vi "basement tank 1.vi"() -> ()   [LabVIEW 2019]
uses:
  <vilib>/NI/Current Value Table/Type Defs/Single Tag.ctl
  <vilib>/NI/Current Value Table/Type Defs/Data Types.ctl
  <vilib>/Utility/miscctls.llb/LVPointTypeDef.ctl
  <vilib>/NI/STM/TCP/Read Meta Data (TCP Ref).vi
  <vilib>/NI/STM/TCP/Get Connection Reference (TCP).vi
  <vilib>/NI/AMC/Read Termination Message.vi
  <vilib>/NI/AMC/Create Single Message.vi
  <vilib>/NI/AMC/Update Message Routing Info.vi
  <vilib>/NI/STM/TCP/Read Meta Data (TCP Clst).vi
  <vilib>/NI/AMC/Globals.vi
  <vilib>/NI/STM/TCP/Write Message (TCP).vi
  <vilib>/NI/AMC/Send Message.vi
  <vilib>/NI/AMC/AMC.lvlib
  <vilib>/NI/STM/NI STM.lvlib
  <vilib>/NI/Current Value Table/Current Value Table.lvlib
panel:
  in  "Auto Level Main Tank":dbl(knob)=250.0 min=250.0 max=950.0 step=1.0 scale=200.0..1000.0 scale format="%#.3g"
  in  "Enable DI Auto Top-up":bool
  in  "Sulfuric Proc 1":dbl=2.0 caption="ml Acid Proc 1" min=0.0 max=5000.0 step=1.0
  in  "Trig Sulfuric Proc1":bool caption="Trigger Dose"
  out "Flow":bool
  in  "LEV Proc 1":dbl=2.0 caption="ml Lev Proc 1" min=0.0 max=1000.0 step=1.0
  in  "Trig Level Proc1":bool caption="Trigger Dose"
  in  "UCON Proc 1":dbl=2.0 caption="ml UCON Proc 1" min=0.0 max=1000.0 step=1.0
  in  "Trig UCON Proc 1":bool caption="Trigger Dose"
  in  "SPS Proc 1":dbl=2.0 caption="ml SPS Proc 1" min=0.0 max=1000.0 step=1.0
  in  "Trig SPS Proc 1":bool caption="Trigger Dose"
  in  "BasT1_Level Last Hr":bool
  in  "BasT1_Flow Last Hr":bool
  in  "Specific Gravity":dbl(knob)=1.0 min=1.0 max=1.25 step=0.0025 scale=1.0..1.25
  in  "CuOAddAmount":dbl caption="CuO grams to add" min=-1000.0 max=1000.0 step=1.0
  out "Grams CuO to Add":dbl format="%.1f"
  in  "Dose Extra Oxide":bool
  out "BTnk1 SG":dbl format="%.3f"
  in  "FlowInd OxSys":dbl(slide) scale=0.0..15.0
  out "Chilled Injection":u8(slide) scale=0.0..100.0
  out "Tempered Injection":u8(slide) scale=0.0..100.0
  in  "BasT1_P Last Hr":bool
  in  "BasT1_T Last Hr":bool
  out "Boiler Water Facilities Valve":dbl(slide) scale=0.0..100.0
  out "Tempered Water Facilities Valve":dbl(slide) scale=0.0..100.0
  out "Chilled Water Facilities Valve":dbl(slide) scale=0.0..100.0
  out "Boiler Water Out":dbl(knob) scale=10.0..110.0
  out "Boiler Water In":dbl(knob) scale=10.0..110.0
  out "Tempered Water Out":dbl(knob) scale=10.0..35.0
  out "Tempered Water In":dbl(knob) scale=10.0..35.0
  out "Chilled Water Out":dbl(knob) scale=0.0..25.0
  out "Chilled Water In":dbl(knob) scale=0.0..25.0
  out "E Stop":bool
  out "OxideToFilter":bool
  out "Oxide Pump":bool
  out "Boolean 4":bool
  out "OxideDose Indicate":bool
  out "To Plating Process 1 & 2":bool
  out "ThreewayLowerElbow":bool
  in  "Tab Control":enum32{"Main Pump", "Lift Pump"}(tab)
  out "Amps":dbl format="%#.2g"
  out "Volts":dbl format="%#.1f"
  out "VFD T":dbl format="%#.2g"
  out "RPM":dbl format="%#.2f"
  out "Fault Code":dbl format="%#.2g"
  out "Freq":dbl format="%#.2g"
  out "PipeToTank":bool
  out "Tnk1Tee 2":bool
  out "Boolean 6":bool
  out "Circulator":bool
  out "Run Enabled?":bool
  out "Supply Pressure (kPa)":dbl(knob) scale=0.0..250.0
  out "Supply Temperature":dbl(slide) scale=0.0..100.0
  in  "Draining System to Tree":bool
  in  "Liters DI to Add":dbl(knob) min=0.0 max=500.0 step=1.0 scale=0.0..500.0
  in  "Add DI Water":bool
  out "PipeToPump 2":bool
  out "Total Added":dbl format="%.2g"
  out "DI Flow (L/min)":dbl(knob) scale=0.0..100.0
  out "Total Flow (when operated with plating tanks)":dbl(knob) scale=0.0..150.0
  in  "Flow to Reactor (L/min)":dbl(knob)=5.0 min=5.0 max=20.0 step=0.1 scale=5.0..12.0 scale format="%#.1g"
  in  "Enable Oxide Reactor":bool
  in  "Enable T-Control":bool
  in  "Temperature Setpoint":dbl(knob) step=0.1 scale=12.0..30.0 scale format="%#.1g"
  in  "Supply Pressure (kPa)":dbl(knob)=50.0 min=50.0 max=200.0 step=5.0 scale=50.0..200.0
  out "HeatExchanger":bool
  out "PipeToPump":bool
  out "Tnk1Tee":bool
  in  "Enable Main Pump":bool
  out "Main Pump":bool
  out "Tank":dbl(slide) scale=0.0..1000.0
  in  "Machine":bool
  in  "Basement 4":bool
  in  "Dryer":bool
  in  "Rinse 4":bool
  in  "Rinse 3":bool
  in  "Rinse 2":bool
  in  "Basement 3":bool
  in  "Basement 2":bool
  in  "Basement 1":bool
  in  "Plater 6":bool
  in  "Plater 5":bool
  in  "Plater 4":bool
  in  "Plater 3":bool
  in  "Plater 2":bool
  in  "Plater 1":bool
  in  "Predip":bool
  in  "Rinse 1":bool
  in  "Cleaner":bool
  in  "Etch":bool
  out "status":string
  # "Module Selection"
  # "@"
  # "SG"
  # "Dosing"
  # "SPS"
  # "UCON"
  # "Leveler"
  # "Sulfuric Acid"
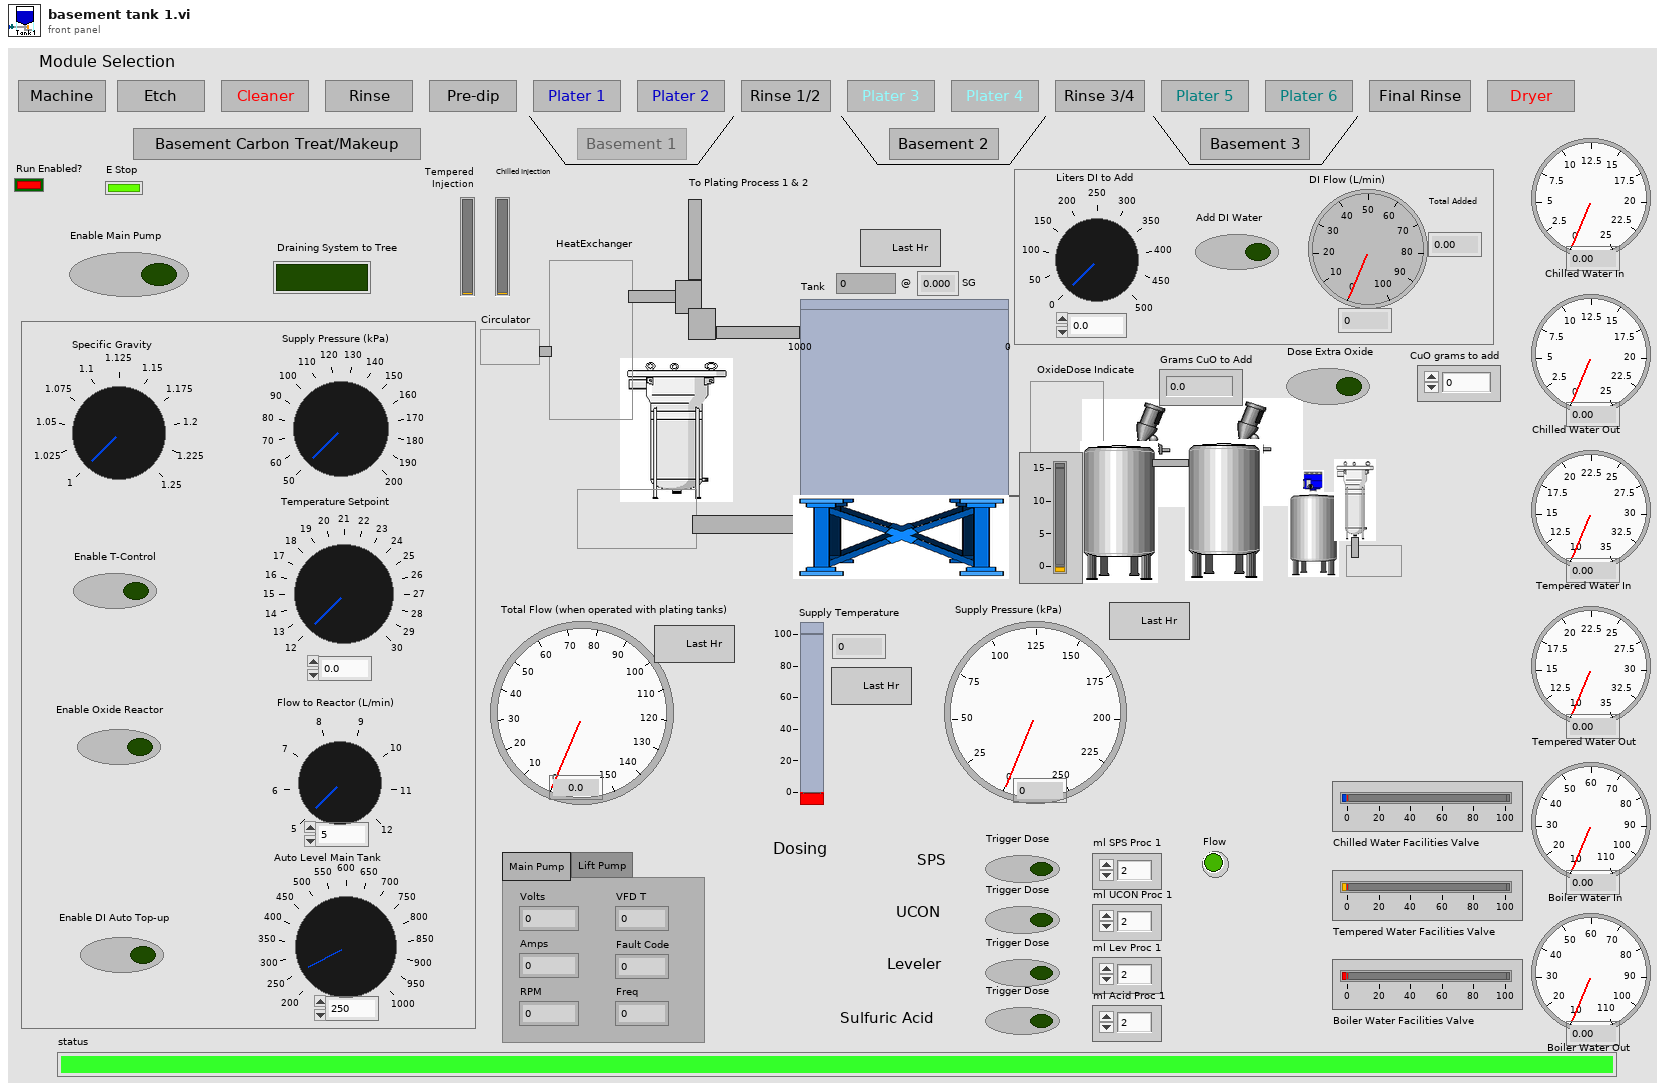
[diagram p1: front panel]
types:
  T1 = typedef "Current Value Table.lvlib/Single Tag.ctl" = cluster{"Data Type":T2, "Name":string, "Value":string, "Description":string}
  T2 = typedef "Current Value Table.lvlib/Data Types.ctl" = enum16{"Double", "Single", "I64", "I32", "I16", "I8", "U64", "U32", "U16", "U8", "String", "Boolean", "Array of U8", "Array of U16", "Array of U32", "Array of U64", "Array of I64", "Array of I32", "Array of I16", "Array of I8", "Array of Double", "Array of Single", "Array of Boolean", "Array of String"}
  T3 = typedef "NI STM.lvlib/TCP Connection Info.ctl" = cluster{"connection ID":refnum<k5>, "meta data":T4[]}
  T4 = typedef "NI STM.lvlib/MetaDataElement.ctl" = string
  T5 = typedef "AMC.lvlib/Message Queue.ctl" = refnum<queue>
  T6 = cluster{"Shift":bool, "Ctrl":bool, "Alt":bool, "Cmd":bool, "Opt":bool}
  T7 = enum8{"Enabled", "Disabled", "Disabled and Grayed Out"}
  T8 = typedef "LVPointTypeDef.ctl" = cluster{"Horizontal":i16, "Vertical":i16}
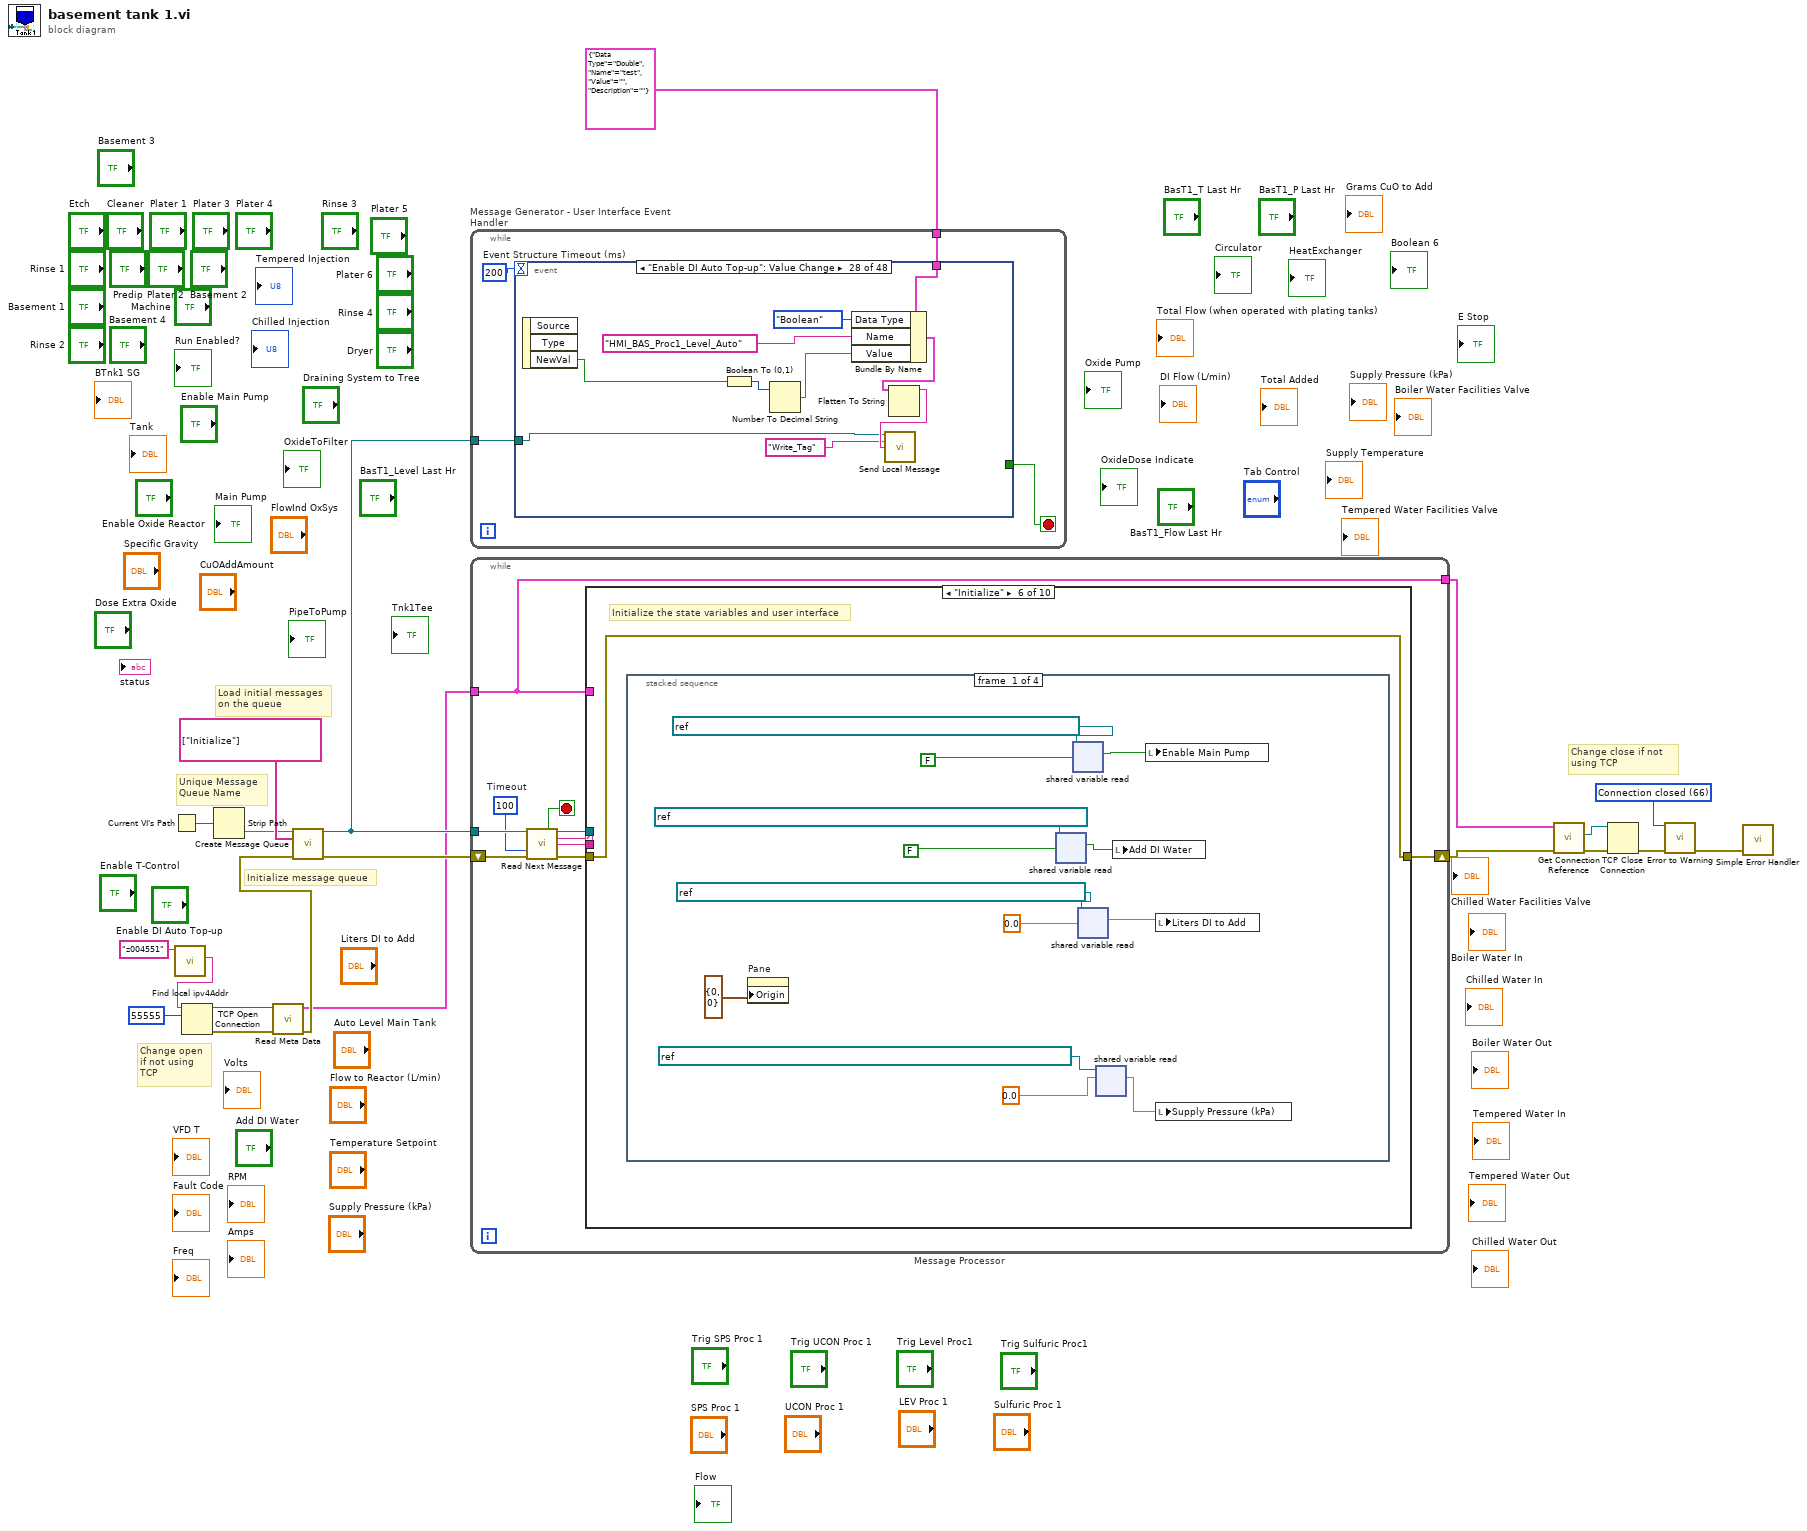
[diagram p0: block diagram]
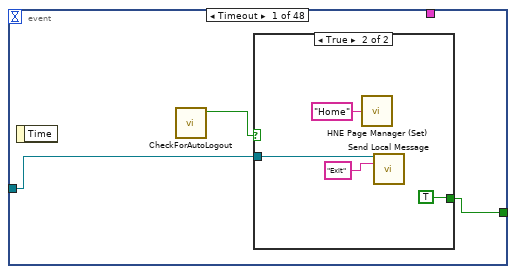
[diagram p2: hidden frame]
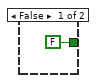
[diagram p3: hidden frame]
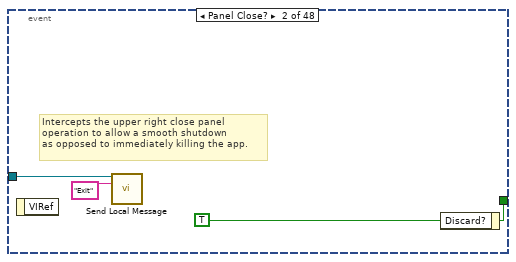
[diagram p4: hidden frame]
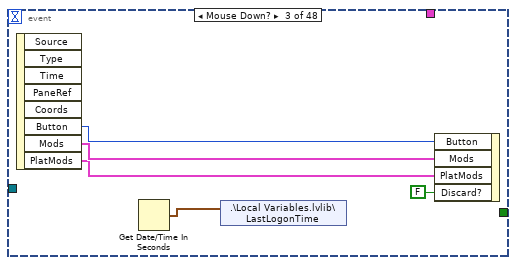
[diagram p5: hidden frame]
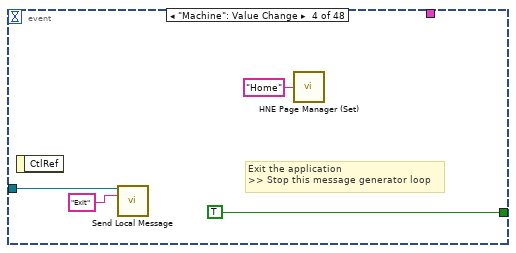
[diagram p6: hidden frame]
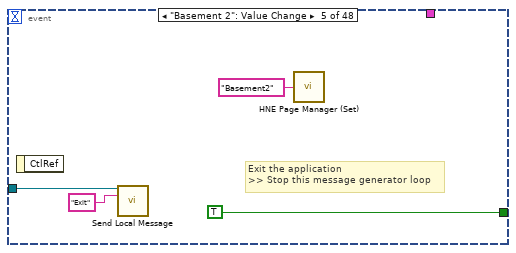
[diagram p7: hidden frame]
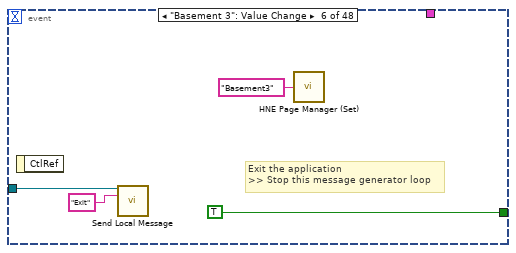
[diagram p8: hidden frame]
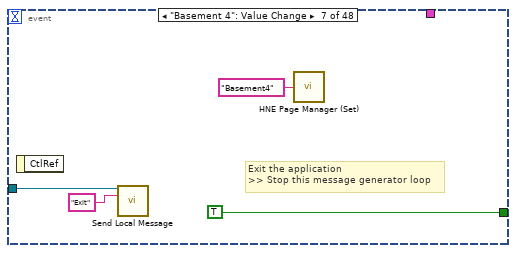
[diagram p9: hidden frame]
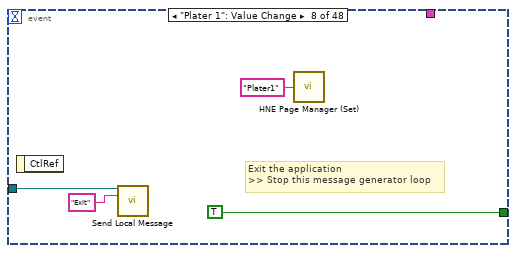
[diagram p10: hidden frame]
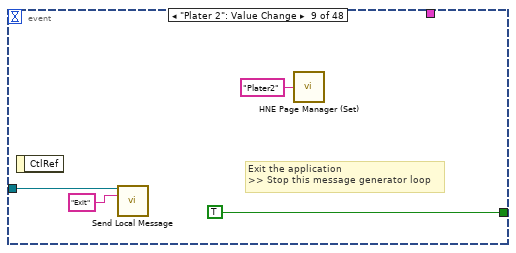
[diagram p11: hidden frame]
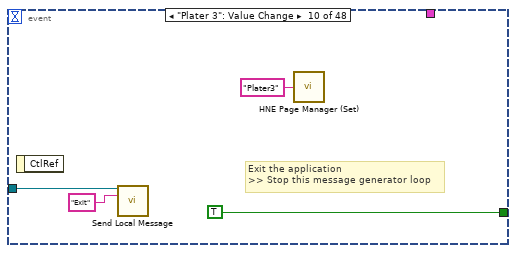
[diagram p12: hidden frame]
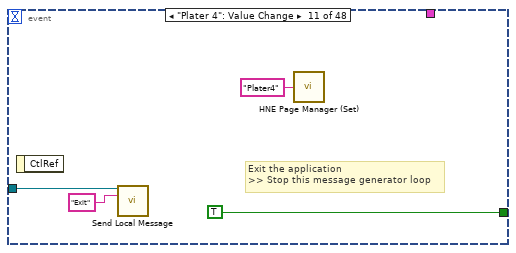
[diagram p13: hidden frame]
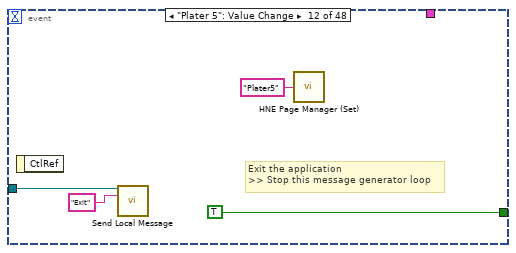
[diagram p14: hidden frame]
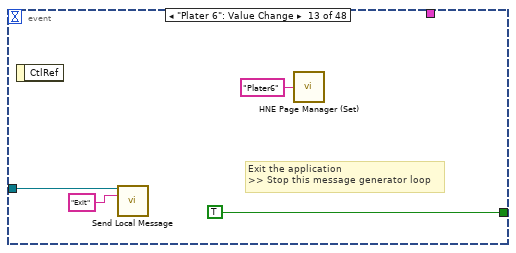
[diagram p15: hidden frame]
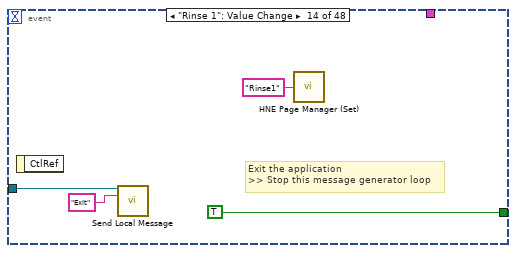
[diagram p16: hidden frame]
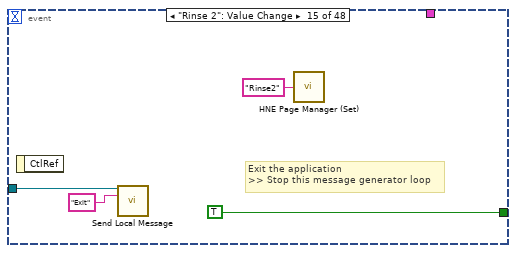
[diagram p17: hidden frame]
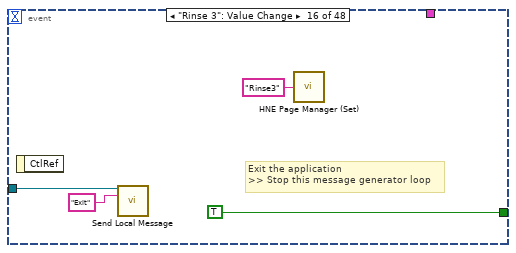
[diagram p18: hidden frame]
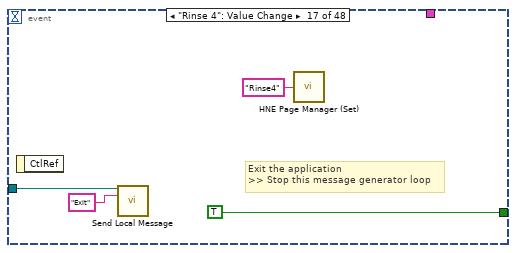
[diagram p19: hidden frame]
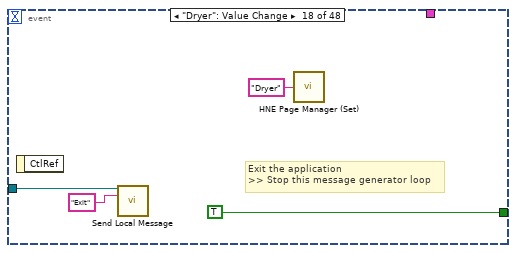
[diagram p20: hidden frame]
diagram:
  w9 = 66 items=["No Error", "Argument Error", "Memory Full", "Out of Zone", "End of File", "File Already Open", "Generic File IO Error", "File Not Found", "File Permission Error", "Disk Full", "Duplicate Path", "Too Many Files Open", "Not Enabled", "Resource File Not Found", "Cannot Add Resource", "Resource Not Found", "Image Not Found", "Image Memory Error", "Pen Does Not Exist", "Config Bad Type", "Config Token Not Found", "Config Parse Error", "Config Memory Error", "Bad External Code Format", "Bad External Code Offset", "External Code Not Present", "Null Window", "Destroy Window Mixup", "Null Menu", "Print Aborted", "Bad Print Record", "Print Driver Error", "Windows Error During Print", "Memory Error During Print", "Print Dialog Error", "Generic Print Error", "Invalid Device Refnum", "Device Not Found", "Device Parameter Error", "Device Unit Error", "Can't Open Device", "Device Call Aborted", "Generic Error", "Cancelled By User", "Object ID Too Low", "Object ID Too High", "Object Not In Heap", "Unknown Heap", "Bad DefProc ID", "DefProc Not In Table", "Message Out Of Range", "Null Method", "Unknown Message", "Manager Call Not Supported", "Bad address", "Connection In progress", "Connection timed out", "Connection is already in progress", "Network attribute not supported", "Network error", "Address in use", "System out of memory", "Connection aborted", "Connection refused", "Connection is not connected", "Connection is already connected", "Connection closed", "Initialize error (interapplication manager)", "Bad occurrence", "Wait on unbound occurrence handler", "Occurrence queue overflow", "Bad path", "Semaphore not signaled", "Unrecognized type (interapplication manager)"] ("1st Error to Convert")
  # "Change close if not using TCP"
  # "Change open if not using TCP"
  # "Initialize message queue"
  # "Unique Message\nQueue Name"
  # "Load initial messages\non the queue"
  n1 = Current VI's Path() -> (path=w16:path)
  n2 = call "Find local ipv4Addr.vi"("MachineToFind"="z004551" ("Target IP Address")) -> ("name"=w1:string)  [unwired: 9 in, 1 out]
  n3 = TCP Open Connection(address=w1, remote port or service name=u16 55555 ("remote port")) -> (connection ID=w14:refnum<k5>, error out=w13:errorcluster)  [unwired: 1 in, 2 out]
  n4 = Strip Path(path=w16) -> (name=w19:string)  [unwired: 1 out]
  n5 = call-poly <vilib>:"Read Meta Data.vi"("error in"=w13, "connection ID"=w14) -> ("error out"=w12:errorcluster, "connection info out"=w11:T3)  [unwired: 7 in, 1 out]
  n6 = call <vilib>:"Create Message Queue.vi"("message queue name"=w19, "initial message names"=string[] ["Initialize"], "error in"=w12) -> ("message queue out"=w18:T5, "error out"=w17:errorcluster)  [unwired: 11 in]
  n7 = while "Message Generator - User Interface Event Handler" {
    tunnel: w18 -> [w22]
    tunnel: T1 {"Data Type"=enum."Double", "Name"="test", "Value"="", "Description"=""} ("Tag") -> [w21]
    stop <- w23 stop-if-true
    w24 = 200  # Event Structure Timeout (ms)
    n8 = event shown="[27] \"Enable DI Auto Top-up\": Value Change" {
      selector: _ -> [_ _ _ _ _ _ _ _ _ _ _ _ _ _ _ _ _ _ _ _ _ _ _ _ _ _ _ _ _ _ _ _ _ _ _ _ _ _ _ _ _ _ _ _ _ _ _ _]
      dyn-events: _ -> [_ _ _ _ _ _ _ _ _ _ _ _ _ _ _ _ _ _ _ _ _ _ _ _ _ _ _ _ _ _ _ _ _ _ _ _ _ _ _ _ _ _ _ _ _ _ _ _]
      timeout: w24 -> [_ _ _ _ _ _ _ _ _ _ _ _ _ _ _ _ _ _ _ _ _ _ _ _ _ _ _ _ _ _ _ _ _ _ _ _ _ _ _ _ _ _ _ _ _ _ _ _]
      tunnel: [w25 w35 _ TRUE ("Discard?") TRUE ("Discard?") TRUE ("Discard?") TRUE ("Discard?") TRUE ("Discard?") TRUE ("Discard?") TRUE ("Discard?") TRUE ("Discard?") TRUE ("Discard?") TRUE ("Discard?") TRUE ("Discard?") TRUE ("Discard?") TRUE ("Discard?") TRUE ("Discard?") TRUE ("Discard?") TRUE ("Discard?") TRUE ("Discard?") TRUE ("Discard?") _ _ _ _ _ _ _ _ _ _ _ _ _ _ _ _ _ _ _ _ _ _ _ _ _ _ _] -> w23
      tunnel: w22 -> [w26 w33 _ w42 w46 w50 w54 w58 w62 w66 w70 w74 w78 w82 w86 w90 w94 w98 w102 w106 w110 w113 w115 w125 w135 w145 w155 w165 w175 w185 w195 w205 w215 w225 w234 w243 w252 w261 w270 w279 w288 w297 w306 w315 w324 w329 w334 w339]
      tunnel: w21 -> [_ _ _ _ _ _ _ _ _ _ _ _ _ _ _ _ _ _ _ _ _ _ w116 w126 w136 w146 w156 w166 w176 w186 w196 w206 w216 w228 w237 w246 w255 w264 w273 w282 w291 w300 w309 w318 _ _ _ _]
      event Timeout {
        n9 = event-data() -> ()  [unwired: 2 out]
        n10 = call "CheckForAutoLogout.vi"() -> ("Boolean"=w27:bool)  [unwired: 11 in]
        n11 = case shown="True" w27 {
          tunnel: [FALSE ("Discard?") TRUE ("Discard?")] -> w25
          tunnel: w26 -> [_ w29]
          frame False {
          }
          frame True {
            n12 = call <userlib>:"HNE Page Manager (Set).vi"("Next Page"="Home") -> ()  [unwired: 4 in, 1 out]
            n13 = call <vilib>:"Send Local Message.vi"("message queue in"=w29, "message name"="Exit") -> ()  [unwired: 11 in, 3 out]
          }
        }
      }
      event Panel Close? {
        w35 = TRUE ("Discard?")
        # "Intercepts the upper right close panel\noperation to allow a smooth shutdown\nas opposed to immediately killing the app."
        n14 = event-data() -> ()  [unwired: 2 out]
        n15 = call <vilib>:"Send Local Message.vi"("message queue in"=w33, "message name"="Exit") -> ()  [unwired: 11 in, 3 out]
        n16 = event-data("Discard?"=w35) -> ()  [unwired: 1 in, 1 out]
      }
      event Mouse Down? {
        n17 = event-data() -> ("Button"=w40:u16, "Mods"=w39:cluster{"Double Click":bool, "Menu Key":bool}, "PlatMods"=w38:T6)  [unwired: 6 out]
        n18 = Get Date/Time In Seconds() -> (seconds since 1Jan1904=w36:timestamp)
        n19 = shared-variable ".\\Local Variables.lvlib\\LastLogonTime"(w36) -> ()  [unwired: 1 in, 1 out]
        n20 = event-data("Button"=w40, "Mods"=w39, "PlatMods"=w38, "Discard?"=FALSE) -> ()  [unwired: 1 in, 1 out]
      }
      event "Machine": Value Change {
        # "Exit the application\n>> Stop this message generator loop"
        n21 = event-data() -> ()  [unwired: 2 out]
        n22 = call <vilib>:"Send Local Message.vi"("message queue in"=w42, "message name"="Exit") -> ()  [unwired: 11 in, 3 out]
        n23 = call <userlib>:"HNE Page Manager (Set).vi"("Next Page"="Home") -> ()  [unwired: 4 in, 1 out]
      }
      event "Basement 2": Value Change {
        # "Exit the application\n>> Stop this message generator loop"
        n24 = event-data() -> ()  [unwired: 2 out]
        n25 = call <vilib>:"Send Local Message.vi"("message queue in"=w46, "message name"="Exit") -> ()  [unwired: 11 in, 3 out]
        n26 = call <userlib>:"HNE Page Manager (Set).vi"("Next Page"="Basement2") -> ()  [unwired: 4 in, 1 out]
      }
      event "Basement 3": Value Change {
        # "Exit the application\n>> Stop this message generator loop"
        n27 = event-data() -> ()  [unwired: 2 out]
        n28 = call <vilib>:"Send Local Message.vi"("message queue in"=w50, "message name"="Exit") -> ()  [unwired: 11 in, 3 out]
        n29 = call <userlib>:"HNE Page Manager (Set).vi"("Next Page"="Basement3") -> ()  [unwired: 4 in, 1 out]
      }
      event "Basement 4": Value Change {
        # "Exit the application\n>> Stop this message generator loop"
        n30 = event-data() -> ()  [unwired: 2 out]
        n31 = call <vilib>:"Send Local Message.vi"("message queue in"=w54, "message name"="Exit") -> ()  [unwired: 11 in, 3 out]
        n32 = call <userlib>:"HNE Page Manager (Set).vi"("Next Page"="Basement4") -> ()  [unwired: 4 in, 1 out]
      }
      event "Plater 1": Value Change {
        # "Exit the application\n>> Stop this message generator loop"
        n33 = event-data() -> ()  [unwired: 2 out]
        n34 = call <vilib>:"Send Local Message.vi"("message queue in"=w58, "message name"="Exit") -> ()  [unwired: 11 in, 3 out]
        n35 = call <userlib>:"HNE Page Manager (Set).vi"("Next Page"="Plater1") -> ()  [unwired: 4 in, 1 out]
      }
      event "Plater 2": Value Change {
        # "Exit the application\n>> Stop this message generator loop"
        n36 = event-data() -> ()  [unwired: 2 out]
        n37 = call <vilib>:"Send Local Message.vi"("message queue in"=w62, "message name"="Exit") -> ()  [unwired: 11 in, 3 out]
        n38 = call <userlib>:"HNE Page Manager (Set).vi"("Next Page"="Plater2") -> ()  [unwired: 4 in, 1 out]
      }
      event "Plater 3": Value Change {
        # "Exit the application\n>> Stop this message generator loop"
        n39 = event-data() -> ()  [unwired: 2 out]
        n40 = call <vilib>:"Send Local Message.vi"("message queue in"=w66, "message name"="Exit") -> ()  [unwired: 11 in, 3 out]
        n41 = call <userlib>:"HNE Page Manager (Set).vi"("Next Page"="Plater3") -> ()  [unwired: 4 in, 1 out]
      }
      event "Plater 4": Value Change {
        # "Exit the application\n>> Stop this message generator loop"
        n42 = event-data() -> ()  [unwired: 2 out]
        n43 = call <vilib>:"Send Local Message.vi"("message queue in"=w70, "message name"="Exit") -> ()  [unwired: 11 in, 3 out]
        n44 = call <userlib>:"HNE Page Manager (Set).vi"("Next Page"="Plater4") -> ()  [unwired: 4 in, 1 out]
      }
      event "Plater 5": Value Change {
        # "Exit the application\n>> Stop this message generator loop"
        n45 = event-data() -> ()  [unwired: 2 out]
        n46 = call <vilib>:"Send Local Message.vi"("message queue in"=w74, "message name"="Exit") -> ()  [unwired: 11 in, 3 out]
        n47 = call <userlib>:"HNE Page Manager (Set).vi"("Next Page"="Plater5") -> ()  [unwired: 4 in, 1 out]
      }
      event "Plater 6": Value Change {
        # "Exit the application\n>> Stop this message generator loop"
        n48 = event-data() -> ()  [unwired: 2 out]
        n49 = call <vilib>:"Send Local Message.vi"("message queue in"=w78, "message name"="Exit") -> ()  [unwired: 11 in, 3 out]
        n50 = call <userlib>:"HNE Page Manager (Set).vi"("Next Page"="Plater6") -> ()  [unwired: 4 in, 1 out]
      }
      event "Rinse 1": Value Change {
        # "Exit the application\n>> Stop this message generator loop"
        n51 = event-data() -> ()  [unwired: 2 out]
        n52 = call <vilib>:"Send Local Message.vi"("message queue in"=w82, "message name"="Exit") -> ()  [unwired: 11 in, 3 out]
        n53 = call <userlib>:"HNE Page Manager (Set).vi"("Next Page"="Rinse1") -> ()  [unwired: 4 in, 1 out]
      }
      event "Rinse 2": Value Change {
        # "Exit the application\n>> Stop this message generator loop"
        n54 = event-data() -> ()  [unwired: 2 out]
        n55 = call <vilib>:"Send Local Message.vi"("message queue in"=w86, "message name"="Exit") -> ()  [unwired: 11 in, 3 out]
        n56 = call <userlib>:"HNE Page Manager (Set).vi"("Next Page"="Rinse2") -> ()  [unwired: 4 in, 1 out]
      }
      event "Rinse 3": Value Change {
        # "Exit the application\n>> Stop this message generator loop"
        n57 = event-data() -> ()  [unwired: 2 out]
        n58 = call <vilib>:"Send Local Message.vi"("message queue in"=w90, "message name"="Exit") -> ()  [unwired: 11 in, 3 out]
        n59 = call <userlib>:"HNE Page Manager (Set).vi"("Next Page"="Rinse3") -> ()  [unwired: 4 in, 1 out]
      }
      event "Rinse 4": Value Change {
        # "Exit the application\n>> Stop this message generator loop"
        n60 = event-data() -> ()  [unwired: 2 out]
        n61 = call <vilib>:"Send Local Message.vi"("message queue in"=w94, "message name"="Exit") -> ()  [unwired: 11 in, 3 out]
        n62 = call <userlib>:"HNE Page Manager (Set).vi"("Next Page"="Rinse4") -> ()  [unwired: 4 in, 1 out]
      }
      event "Dryer": Value Change {
        # "Exit the application\n>> Stop this message generator loop"
        n63 = event-data() -> ()  [unwired: 2 out]
        n64 = call <vilib>:"Send Local Message.vi"("message queue in"=w98, "message name"="Exit") -> ()  [unwired: 11 in, 3 out]
        n65 = call <userlib>:"HNE Page Manager (Set).vi"("Next Page"="Dryer") -> ()  [unwired: 4 in, 1 out]
      }
      event "Predip": Value Change {
        # "Exit the application\n>> Stop this message generator loop"
        n66 = event-data() -> ()  [unwired: 2 out]
        n67 = call <vilib>:"Send Local Message.vi"("message queue in"=w102, "message name"="Exit") -> ()  [unwired: 11 in, 3 out]
        n68 = call <userlib>:"HNE Page Manager (Set).vi"("Next Page"="Predip") -> ()  [unwired: 4 in, 1 out]
      }
      event "Cleaner": Value Change {
        # "Exit the application\n>> Stop this message generator loop"
        n69 = event-data() -> ()  [unwired: 2 out]
        n70 = call <vilib>:"Send Local Message.vi"("message queue in"=w106, "message name"="Exit") -> ()  [unwired: 11 in, 3 out]
        n71 = call <userlib>:"HNE Page Manager (Set).vi"("Next Page"="Clean") -> ()  [unwired: 4 in, 1 out]
      }
      event "Etch": Value Change {
        # "Exit the application\n>> Stop this message generator loop"
        n72 = event-data() -> ()  [unwired: 2 out]
        n73 = call <vilib>:"Send Local Message.vi"("message queue in"=w110, "message name"="Exit") -> ()  [unwired: 11 in, 3 out]
        n74 = call <userlib>:"HNE Page Manager (Set).vi"("Next Page"="Etch") -> ()  [unwired: 4 in, 1 out]
      }
      event Menu Selection (User) {
        # "Add run-time menu items to the message\nqueue. The message handler case names must match the menu ItemTag names."
        n75 = event-data() -> ("ItemTag"=w114:string)  [unwired: 1 out]
        n76 = call <vilib>:"Send Local Message.vi"("message queue in"=w113, "message name"=w114) -> ()  [unwired: 11 in, 3 out]
      }
      event "Enable Main Pump": Value Change {
        n77 = event-data() -> ("NewVal"=w117:bool)  [unwired: 3 out]
        n78 = Boolean To (0,1)(Boolean=w117) -> (0, 1=w124:i16)
        n79 = Number To Decimal String(number=w124) -> (decimal integer string=w123:string)  [unwired: 1 in]
        n80 = Bundle By Name(cluster=w116, "Data Type"=Data_Types."Boolean", "Name"="HMI_Enable_BTnk1_Pump", "Value"=w123) -> (w122:T1)
        n81 = Flatten To String(anything=w122) -> (data string=w121:string)  [unwired: 3 in, 2 out]
        n82 = call <vilib>:"Send Local Message.vi"("message queue in"=w115, "message name"="Write_Tag", "message value"=w121) -> ()  [unwired: 10 in, 3 out]
      }
      event "Enable T-Control": Value Change {
        n83 = event-data() -> ("NewVal"=w127:bool)  [unwired: 3 out]
        n84 = Boolean To (0,1)(Boolean=w127) -> (0, 1=w134:i16)
        n85 = Number To Decimal String(number=w134) -> (decimal integer string=w133:string)  [unwired: 1 in]
        n86 = Bundle By Name(cluster=w126, "Data Type"=Data_Types."Boolean", "Name"="HMI_BAS_Tank1_TControl_Enable", "Value"=w133) -> (w132:T1)
        n87 = Flatten To String(anything=w132) -> (data string=w131:string)  [unwired: 3 in, 2 out]
        n88 = call <vilib>:"Send Local Message.vi"("message queue in"=w125, "message name"="Write_Tag", "message value"=w131) -> ()  [unwired: 10 in, 3 out]
      }
      event "Enable Oxide Reactor": Value Change {
        n89 = event-data() -> ("NewVal"=w137:bool)  [unwired: 3 out]
        n90 = Boolean To (0,1)(Boolean=w137) -> (0, 1=w144:i16)
        n91 = Number To Decimal String(number=w144) -> (decimal integer string=w143:string)  [unwired: 1 in]
        n92 = Bundle By Name(cluster=w136, "Data Type"=Data_Types."Boolean", "Name"="HMI_Proc1_Run_OxideSys", "Value"=w143) -> (w142:T1)
        n93 = Flatten To String(anything=w142) -> (data string=w141:string)  [unwired: 3 in, 2 out]
        n94 = call <vilib>:"Send Local Message.vi"("message queue in"=w135, "message name"="Write_Tag", "message value"=w141) -> ()  [unwired: 10 in, 3 out]
      }
      event "Draining System to Tree": Value Change {
        n95 = event-data() -> ("NewVal"=w147:bool)  [unwired: 3 out]
        n96 = Boolean To (0,1)(Boolean=w147) -> (0, 1=w154:i16)
        n97 = Number To Decimal String(number=w154) -> (decimal integer string=w153:string)  [unwired: 1 in]
        n98 = Bundle By Name(cluster=w146, "Data Type"=Data_Types."Boolean", "Name"="HMI_Drain_BTank1", "Value"=w153) -> (w152:T1)
        n99 = Flatten To String(anything=w152) -> (data string=w151:string)  [unwired: 3 in, 2 out]
        n100 = call <vilib>:"Send Local Message.vi"("message queue in"=w145, "message name"="Write_Tag", "message value"=w151) -> ()  [unwired: 10 in, 3 out]
      }
      event "Add DI Water": Value Change {
        n101 = event-data() -> ("NewVal"=w157:bool)  [unwired: 3 out]
        n102 = Boolean To (0,1)(Boolean=w157) -> (0, 1=w164:i16)
        n103 = Number To Decimal String(number=w164) -> (decimal integer string=w163:string)  [unwired: 1 in]
        n104 = Bundle By Name(cluster=w156, "Data Type"=Data_Types."Boolean", "Name"="HMI_BAS_Proc1_AddDIVolume", "Value"=w163) -> (w162:T1)
        n105 = Flatten To String(anything=w162) -> (data string=w161:string)  [unwired: 3 in, 2 out]
        n106 = call <vilib>:"Send Local Message.vi"("message queue in"=w155, "message name"="Write_Tag", "message value"=w161) -> ()  [unwired: 10 in, 3 out]
      }
      event "Enable DI Auto Top-up": Value Change {
        n107 = event-data() -> ("NewVal"=w167:bool)  [unwired: 3 out]
        n108 = Boolean To (0,1)(Boolean=w167) -> (0, 1=w174:i16)
        n109 = Number To Decimal String(number=w174) -> (decimal integer string=w173:string)  [unwired: 1 in]
        n110 = Bundle By Name(cluster=w166, "Data Type"=Data_Types."Boolean", "Name"="HMI_BAS_Proc1_Level_Auto", "Value"=w173) -> (w172:T1)
        n111 = Flatten To String(anything=w172) -> (data string=w171:string)  [unwired: 3 in, 2 out]
        n112 = call <vilib>:"Send Local Message.vi"("message queue in"=w165, "message name"="Write_Tag", "message value"=w171) -> ()  [unwired: 10 in, 3 out]
      }
      event "Dose Extra Oxide": Value Change {
        n113 = event-data() -> ("NewVal"=w177:bool)  [unwired: 3 out]
        n114 = Boolean To (0,1)(Boolean=w177) -> (0, 1=w184:i16)
        n115 = Number To Decimal String(number=w184) -> (decimal integer string=w183:string)  [unwired: 1 in]
        n116 = Bundle By Name(cluster=w176, "Data Type"=Data_Types."Boolean", "Name"="HMI_Proc1_Add_CuOxide", "Value"=w183) -> (w182:T1)
        n117 = Flatten To String(anything=w182) -> (data string=w181:string)  [unwired: 3 in, 2 out]
        n118 = call <vilib>:"Send Local Message.vi"("message queue in"=w175, "message name"="Write_Tag", "message value"=w181) -> ()  [unwired: 10 in, 3 out]
      }
      event "Trig SPS Proc 1": Value Change {
        n119 = event-data() -> ("NewVal"=w187:bool)  [unwired: 3 out]
        n120 = Boolean To (0,1)(Boolean=w187) -> (0, 1=w194:i16)
        n121 = Number To Decimal String(number=w194) -> (decimal integer string=w193:string)  [unwired: 1 in]
        n122 = Bundle By Name(cluster=w186, "Data Type"=Data_Types."Boolean", "Name"="HMI_Dose_SPS_Proc1", "Value"=w193) -> (w192:T1)
        n123 = Flatten To String(anything=w192) -> (data string=w191:string)  [unwired: 3 in, 2 out]
        n124 = call <vilib>:"Send Local Message.vi"("message queue in"=w185, "message name"="Write_Tag", "message value"=w191) -> ()  [unwired: 10 in, 3 out]
      }
      event "Trig UCON Proc 1": Value Change {
        n125 = event-data() -> ("NewVal"=w197:bool)  [unwired: 3 out]
        n126 = Boolean To (0,1)(Boolean=w197) -> (0, 1=w204:i16)
        n127 = Number To Decimal String(number=w204) -> (decimal integer string=w203:string)  [unwired: 1 in]
        n128 = Bundle By Name(cluster=w196, "Data Type"=Data_Types."Boolean", "Name"="HMI_Dose_UCON_Proc1", "Value"=w203) -> (w202:T1)
        n129 = Flatten To String(anything=w202) -> (data string=w201:string)  [unwired: 3 in, 2 out]
        n130 = call <vilib>:"Send Local Message.vi"("message queue in"=w195, "message name"="Write_Tag", "message value"=w201) -> ()  [unwired: 10 in, 3 out]
      }
      event "Trig Level Proc1": Value Change {
        n131 = event-data() -> ("NewVal"=w207:bool)  [unwired: 3 out]
        n132 = Boolean To (0,1)(Boolean=w207) -> (0, 1=w214:i16)
        n133 = Number To Decimal String(number=w214) -> (decimal integer string=w213:string)  [unwired: 1 in]
        n134 = Bundle By Name(cluster=w206, "Data Type"=Data_Types."Boolean", "Name"="HMI_Dose_Leveler_Proc1", "Value"=w213) -> (w212:T1)
        n135 = Flatten To String(anything=w212) -> (data string=w211:string)  [unwired: 3 in, 2 out]
        n136 = call <vilib>:"Send Local Message.vi"("message queue in"=w205, "message name"="Write_Tag", "message value"=w211) -> ()  [unwired: 10 in, 3 out]
      }
      event "Trig Sulfuric Proc1": Value Change {
        n137 = event-data() -> ("NewVal"=w217:bool)  [unwired: 3 out]
        n138 = Boolean To (0,1)(Boolean=w217) -> (0, 1=w224:i16)
        n139 = Number To Decimal String(number=w224) -> (decimal integer string=w223:string)  [unwired: 1 in]
        n140 = Bundle By Name(cluster=w216, "Data Type"=Data_Types."Boolean", "Name"="HMI_Dose_Acid_Proc1", "Value"=w223) -> (w222:T1)
        n141 = Flatten To String(anything=w222) -> (data string=w221:string)  [unwired: 3 in, 2 out]
        n142 = call <vilib>:"Send Local Message.vi"("message queue in"=w215, "message name"="Write_Tag", "message value"=w221) -> ()  [unwired: 10 in, 3 out]
      }
      event "Liters DI to Add": Value Change {
        n143 = event-data() -> ("NewVal"=w227:dbl)  [unwired: 6 out]
        n144 = Number To Fractional String(number=w227) -> (F-format string=w226:string)  [unwired: 3 in]
        n145 = Bundle By Name(cluster=w228, "Data Type"=Data_Types."Double", "Name"="HMI_BAS_Proc1_DI_Setpnt", "Value"=w226) -> (w233:T1)
        n146 = Flatten To String(anything=w233) -> (data string=w232:string)  [unwired: 3 in, 2 out]
        n147 = call <vilib>:"Send Local Message.vi"("message queue in"=w225, "message name"="Write_Tag", "message value"=w232) -> ()  [unwired: 10 in, 3 out]
      }
      event "Auto Level Main Tank": Value Change {
        n148 = event-data() -> ("NewVal"=w236:dbl)  [unwired: 6 out]
        n149 = Number To Fractional String(number=w236) -> (F-format string=w235:string)  [unwired: 3 in]
        n150 = Bundle By Name(cluster=w237, "Data Type"=Data_Types."Double", "Name"="HMI_BAS_Proc1_Level_Setpnt", "Value"=w235) -> (w242:T1)
        n151 = Flatten To String(anything=w242) -> (data string=w241:string)  [unwired: 3 in, 2 out]
        n152 = call <vilib>:"Send Local Message.vi"("message queue in"=w234, "message name"="Write_Tag", "message value"=w241) -> ()  [unwired: 10 in, 3 out]
      }
      event "Flow to Reactor (L/min)": Value Change {
        n153 = event-data() -> ("NewVal"=w245:dbl)  [unwired: 6 out]
        n154 = Number To Fractional String(number=w245) -> (F-format string=w244:string)  [unwired: 3 in]
        n155 = Bundle By Name(cluster=w246, "Data Type"=Data_Types."Double", "Name"="HMI_Proc1_OxFlow_SetPnt", "Value"=w244) -> (w251:T1)
        n156 = Flatten To String(anything=w251) -> (data string=w250:string)  [unwired: 3 in, 2 out]
        n157 = call <vilib>:"Send Local Message.vi"("message queue in"=w243, "message name"="Write_Tag", "message value"=w250) -> ()  [unwired: 10 in, 3 out]
      }
      event "Supply Pressure (kPa)": Value Change {
        n158 = event-data() -> ("NewVal"=w254:dbl)  [unwired: 6 out]
        n159 = Number To Fractional String(number=w254) -> (F-format string=w253:string)  [unwired: 3 in]
        n160 = Bundle By Name(cluster=w255, "Data Type"=Data_Types."Double", "Name"="HMI_BAS_TNK1_P_Setpoint", "Value"=w253) -> (w260:T1)
        n161 = Flatten To String(anything=w260) -> (data string=w259:string)  [unwired: 3 in, 2 out]
        n162 = call <vilib>:"Send Local Message.vi"("message queue in"=w252, "message name"="Write_Tag", "message value"=w259) -> ()  [unwired: 10 in, 3 out]
      }
      event "Temperature Setpoint": Value Change {
        n163 = event-data() -> ("NewVal"=w263:dbl)  [unwired: 6 out]
        n164 = Number To Fractional String(number=w263) -> (F-format string=w262:string)  [unwired: 3 in]
        n165 = Bundle By Name(cluster=w264, "Data Type"=Data_Types."Double", "Name"="HMI_BAS_TNK1_T_Setpoint", "Value"=w262) -> (w269:T1)
        n166 = Flatten To String(anything=w269) -> (data string=w268:string)  [unwired: 3 in, 2 out]
        n167 = call <vilib>:"Send Local Message.vi"("message queue in"=w261, "message name"="Write_Tag", "message value"=w268) -> ()  [unwired: 10 in, 3 out]
      }
      event "Specific Gravity": Value Change {
        n168 = event-data() -> ("NewVal"=w272:dbl)  [unwired: 6 out]
        n169 = Number To Fractional String(number=w272) -> (F-format string=w271:string)  [unwired: 3 in]
        n170 = Bundle By Name(cluster=w273, "Data Type"=Data_Types."Double", "Name"="HMI_BAS_Proc1_Tank_SG", "Value"=w271) -> (w278:T1)
        n171 = Flatten To String(anything=w278) -> (data string=w277:string)  [unwired: 3 in, 2 out]
        n172 = call <vilib>:"Send Local Message.vi"("message queue in"=w270, "message name"="Write_Tag", "message value"=w277) -> ()  [unwired: 10 in, 3 out]
      }
      event "CuOAddAmount": Value Change {
        n173 = event-data() -> ("NewVal"=w281:dbl)  [unwired: 6 out]
        n174 = Number To Fractional String(number=w281) -> (F-format string=w280:string)  [unwired: 3 in]
        n175 = Bundle By Name(cluster=w282, "Data Type"=Data_Types."Double", "Name"="HMI_Proc1_CuOxideAddAmnt", "Value"=w280) -> (w287:T1)
        n176 = Flatten To String(anything=w287) -> (data string=w286:string)  [unwired: 3 in, 2 out]
        n177 = call <vilib>:"Send Local Message.vi"("message queue in"=w279, "message name"="Write_Tag", "message value"=w286) -> ()  [unwired: 10 in, 3 out]
      }
      event "SPS Proc 1": Value Change {
        n178 = event-data() -> ("NewVal"=w290:dbl)  [unwired: 6 out]
        n179 = Number To Fractional String(number=w290) -> (F-format string=w289:string)  [unwired: 3 in]
        n180 = Bundle By Name(cluster=w291, "Data Type"=Data_Types."Double", "Name"="HMI_SPS_Amount_Proc1", "Value"=w289) -> (w296:T1)
        n181 = Flatten To String(anything=w296) -> (data string=w295:string)  [unwired: 3 in, 2 out]
        n182 = call <vilib>:"Send Local Message.vi"("message queue in"=w288, "message name"="Write_Tag", "message value"=w295) -> ()  [unwired: 10 in, 3 out]
      }
      event "UCON Proc 1": Value Change {
        n183 = event-data() -> ("NewVal"=w299:dbl)  [unwired: 6 out]
        n184 = Number To Fractional String(number=w299) -> (F-format string=w298:string)  [unwired: 3 in]
        n185 = Bundle By Name(cluster=w300, "Data Type"=Data_Types."Double", "Name"="HMI_UCON_Amount_Proc1", "Value"=w298) -> (w305:T1)
        n186 = Flatten To String(anything=w305) -> (data string=w304:string)  [unwired: 3 in, 2 out]
        n187 = call <vilib>:"Send Local Message.vi"("message queue in"=w297, "message name"="Write_Tag", "message value"=w304) -> ()  [unwired: 10 in, 3 out]
      }
      event "LEV Proc 1": Value Change {
        n188 = event-data() -> ("NewVal"=w308:dbl)  [unwired: 6 out]
        n189 = Number To Fractional String(number=w308) -> (F-format string=w307:string)  [unwired: 3 in]
        n190 = Bundle By Name(cluster=w309, "Data Type"=Data_Types."Double", "Name"="HMI_Leveler_Amount_Proc1", "Value"=w307) -> (w314:T1)
        n191 = Flatten To String(anything=w314) -> (data string=w313:string)  [unwired: 3 in, 2 out]
        n192 = call <vilib>:"Send Local Message.vi"("message queue in"=w306, "message name"="Write_Tag", "message value"=w313) -> ()  [unwired: 10 in, 3 out]
      }
      event "Sulfuric Proc 1": Value Change {
        n193 = event-data() -> ("NewVal"=w317:dbl)  [unwired: 6 out]
        n194 = Number To Fractional String(number=w317) -> (F-format string=w316:string)  [unwired: 3 in]
        n195 = Bundle By Name(cluster=w318, "Data Type"=Data_Types."Double", "Name"="HMI_Acid_Amount_Proc1", "Value"=w316) -> (w323:T1)
        n196 = Flatten To String(anything=w323) -> (data string=w322:string)  [unwired: 3 in, 2 out]
        n197 = call <vilib>:"Send Local Message.vi"("message queue in"=w315, "message name"="Write_Tag", "message value"=w322) -> ()  [unwired: 10 in, 3 out]
      }
      event "BasT1_T Last Hr": Value Change {
        n198 = event-data() -> ("NewVal"=w325:bool)  [unwired: 6 out]
        n199 = case shown="True" w325 {
          tunnel: w324 -> [_ w328]
          frame False {
          }
          frame True {
            n200 = call <vilib>:"Send Local Message.vi"("message queue in"=w328, "message name"="DisplayLastHr", "message value"="BAS_Proc1_T") -> ()  [unwired: 10 in, 3 out]
          }
        }
      }
      event "BasT1_P Last Hr": Value Change {
        n201 = event-data() -> ("NewVal"=w330:bool)  [unwired: 6 out]
        n202 = case shown="True" w330 {
          tunnel: w329 -> [_ w333]
          frame False {
          }
          frame True {
            n203 = call <vilib>:"Send Local Message.vi"("message queue in"=w333, "message name"="DisplayLastHr", "message value"="BAS_Proc1_P") -> ()  [unwired: 10 in, 3 out]
          }
        }
      }
      event "BasT1_Flow Last Hr": Value Change {
        n204 = event-data() -> ("NewVal"=w335:bool)  [unwired: 6 out]
        n205 = case shown="True" w335 {
          tunnel: w334 -> [_ w338]
          frame False {
          }
          frame True {
            n206 = call <vilib>:"Send Local Message.vi"("message queue in"=w338, "message name"="DisplayLastHr", "message value"="BAS_Proc1_Total_Flow") -> ()  [unwired: 10 in, 3 out]
          }
        }
      }
      event "BasT1_Level Last Hr": Value Change {
        n207 = event-data() -> ("NewVal"=w340:bool)  [unwired: 6 out]
        n208 = case shown="True" w340 {
          tunnel: w339 -> [_ w343]
          frame False {
          }
          frame True {
            n209 = call <vilib>:"Send Local Message.vi"("message queue in"=w343, "message name"="DisplayLastHr", "message value"="BAS_Proc1_Tank_Level") -> ()  [unwired: 10 in, 3 out]
          }
        }
      }
    }
  }
  n210 = while "Message Processor" {
    shift-left: w17 -> [w349]
    shift-right: [w353] -> w4
    tunnel: w18 -> [w350]
    tunnel: w11 -> [w344]
    tunnel: [w344] -> w5
    stop <- w352 stop-if-true
    w345 = 100  # Timeout
    n211 = call <vilib>:"Read Next Message.vi"("message queue in"=w350, "timeout (1 ms)"=w345, "error in"=w349) -> ("exit process?"=w352:bool, "message queue out"=w351:T5, "message name"=w347:string, "message value"=w346:string, "error out"=w348:errorcluster)  [unwired: 5 in, 3 out]
    n212 = case shown="\"Initialize\"" w347 {
      selector: w347 -> [_ _ w418 _ _ _ _ _ _ _]
      tunnel: w351 -> [_ _ _ _ _ _ w486 _ _ _]
      tunnel: w348 -> [w354 w357 w419 w420 w422 w423 w487 w489 w493 w495]
      tunnel: [w354 w357 w419 errorcluster {"status"=FALSE, "code"=0, "source"=""} ("error out") w422 w423 w485 w489 w492 w495] -> w353
      tunnel: w346 -> [_ _ _ _ _ _ _ _ w491 w496]
      tunnel: w344 -> [_ _ _ _ _ _ _ _ w490 _]
      frame "---------- Framework Operations ----------" {
        # "Dummy case to add a seperator in the Case Structure menu"
      }
      frame "", "Idle" {
        n213 = stacked-sequence {
          frame #0 {
            n214 = control-ref of="status"() -> (w363:refnum<vi>)
            n215 = call <userlib>:"TAE Format Alarm Ticker.vi"("Alarm Ticker Ref"=w363) -> ()  [unwired: 15 in]
            n216 = shared-variable-read(refnum<k21> "ni.var.psp://z004551/CDL0100 ReadWriteTags/HMI_Drain_BTank1" ("shared variable refnum in"), FALSE) -> (w360:bool)  [unwired: 1 in, 3 out]
            n217 = case shown="True" w360 {
              tunnel: [T7."Enabled" ("Disabled") T7."Disabled and Grayed Out" ("Disabled")] -> w359
              frame False {
              }
              frame True {
              }
            }
            n218 = control-ref of="Enable Main Pump"() -> (w358:refnum<vi>)
            n219 = property class="Bool (strict)"(reference=w358, "DisabledEnum"=w359) -> ()  [unwired: 1 in, 2 out]
          }
          frame #1 {
            n220 = shared-variable-read(refnum<k21> "ni.var.psp://z004551/CDL0100 ReadTags/IO_Bas_Tnk1_3Way_At_Recirc" ("shared variable refnum in"), FALSE) -> (w367:bool)  [unwired: 1 in, 3 out]
            n221 = shared-variable-read(refnum<k21> "ni.var.psp://z004551/CDL0100 ReadTags/IO_Bas_Tnk1_3Way_At_Open" ("shared variable refnum in"), FALSE) -> (w370:bool)  [unwired: 1 in, 3 out]
            n222 = shared-variable-read(refnum<k21> "ni.var.psp://z004551/CDL0100 ReadTags/IO_Bas_Tnk1_3Way_At_Closed" ("shared variable refnum in"), FALSE) -> (w373:bool)  [unwired: 1 in, 3 out]
            n223 = Or(x=w370, y=w367) -> (x .or. y?=→"ThreewayLowerElbow" →"PipeToTank":bool)
            n224 = Or(x=w373, y=w370) -> (x .or. y?=w368:bool)
            "To Plating Process 1 & 2" <- w368
            n225 = Or(x=w368, y=w367) -> (x .or. y?=→"Tnk1Tee 2" →"PipeToPump 2":bool)
          }
          frame #2 {
            n226 = control-ref of="Trig SPS Proc 1"() -> (w378:refnum<vi>)
            n227 = shared-variable-read(refnum<k21> "ni.var.psp://z004551/CDL0100 ReadWriteTags/HMI_BAS_Proc1_AddDIVolume" ("shared variable refnum in"), FALSE) -> (w384:bool)  [unwired: 1 in, 3 out]
            n228 = shared-variable-read(refnum<k21> "ni.var.psp://z004551/CDL0100 ReadWriteTags/HMI_Dose_SPS_Proc1" ("shared variable refnum in"), FALSE) -> (w380:bool)  [unwired: 1 in, 3 out]
            n229 = call <userlib>:"Boolean Trigger__ogtk.vi"("Boolean Input"=w380) -> ("Falling Edge"=w379:bool)  [unwired: 1 in, 1 out]
            n230 = call <userlib>:"Boolean Trigger__ogtk.vi"("Boolean Input"=w384) -> ("Falling Edge"=w383:bool)  [unwired: 1 in, 1 out]
            n231 = case shown="True" w379 {
              tunnel: w378 -> [_ w388]
              frame False {
              }
              frame True {
                n232 = property class="Bool (strict)"(reference=w388, "Value"=FALSE) -> ()  [unwired: 1 in, 2 out]
              }
            }
            n233 = case shown="True" w383 {
              frame False {
              }
              frame True {
                n234 = local write "Add DI Water"(FALSE) -> ()
              }
            }
          }
          frame #3 {
            n235 = control-ref of="Trig Level Proc1"() -> (w390:refnum<vi>)
            n236 = control-ref of="Trig UCON Proc 1"() -> (w395:refnum<vi>)
            n237 = shared-variable-read(refnum<k21> "ni.var.psp://z004551/CDL0100 ReadWriteTags/HMI_Dose_UCON_Proc1" ("shared variable refnum in"), FALSE) -> (w397:bool)  [unwired: 1 in, 3 out]
            n238 = shared-variable-read(refnum<k21> "ni.var.psp://z004551/CDL0100 ReadWriteTags/HMI_Dose_Leveler_Proc1" ("shared variable refnum in"), FALSE) -> (w392:bool)  [unwired: 1 in, 3 out]
            n239 = call <userlib>:"Boolean Trigger__ogtk.vi"("Boolean Input"=w397) -> ("Falling Edge"=w396:bool)  [unwired: 1 in, 1 out]
            n240 = call <userlib>:"Boolean Trigger__ogtk.vi"("Boolean Input"=w392) -> ("Falling Edge"=w391:bool)  [unwired: 1 in, 1 out]
            n241 = case shown="True" w396 {
              tunnel: w395 -> [_ w403]
              frame False {
              }
              frame True {
                n242 = property class="Bool (strict)"(reference=w403, "Value"=FALSE) -> ()  [unwired: 1 in, 2 out]
              }
            }
            n243 = case shown="True" w391 {
              tunnel: w390 -> [_ w401]
              frame False {
              }
              frame True {
                n244 = property class="Bool (strict)"(reference=w401, "Value"=FALSE) -> ()  [unwired: 1 in, 2 out]
              }
            }
          }
          frame #4 {
            n245 = control-ref of="Trig Sulfuric Proc1"() -> (w409:refnum<vi>)
            n246 = shared-variable-read(refnum<k21> "ni.var.psp://z004551/CDL0100 ReadWriteTags/HMI_Dose_Acid_Proc1" ("shared variable refnum in"), FALSE) -> (w411:bool)  [unwired: 1 in, 3 out]
            n247 = shared-variable-read(refnum<k21> "ni.var.psp://z004551/CDL0100 ReadTags/BAS_Proc1_Oxide_FlowRate" ("shared variable refnum in"), 0.0) -> (w406:dbl)  [unwired: 1 in, 3 out]
            n248 = call <userlib>:"Boolean Trigger__ogtk.vi"("Boolean Input"=w411) -> ("Falling Edge"=w410:bool)  [unwired: 1 in, 1 out]
            n249 = Greater?(x=w406, y=1.0) -> (0:→"Boolean 4":bool)
            n250 = case shown="True" w410 {
              tunnel: w409 -> [_ w415]
              frame False {
              }
              frame True {
                n251 = property class="Bool (strict)"(reference=w415, "Value"=FALSE) -> ()  [unwired: 1 in, 2 out]
              }
            }
          }
        }
        n252 = shared-variable-read(refnum<k21> "ni.var.psp://z004551/CDL0100 ReadWriteTags/HMI_Enable_BTnk1_Pump" ("shared variable refnum in"), FALSE) -> ()  [unwired: 1 in, 4 out]
      }
      frame "Missing Message Handler", Default {
        # "Call this case if a message is received that is not handled \nby any other case. Typically this is a programming error\nas a result of a typo or unhandled message/missing message handler."
        n253 = Format Into String(format string="DevError: Missing message handler for '%s\" message." ("message"), w418) -> (resulting string=w416:string)  [unwired: 2 in, 1 out]
        n254 = One Button Dialog(message=w416) -> ()  [unwired: 2 out]
      }
      frame "Error" {
        # "General Error Case - this case is called if an error is passed using the error cluster below. Typically most new errors should be handed in each individual case and not passed in the rror cluster. If necessary a custom error handler case should be added and called from other cases."
        n255 = call <vilib>:"Simple Error Handler.vi"("error in (no error)"=w420) -> ()  [unwired: 1 in, 8 out]
      }
      frame "---------- Generic Operations ----------" {
        # "Dummy case to add a seperator in the Case Structure menu"
      }
      frame "Initialize" {
        # "Initialize the state variables and user interface"
        n256 = stacked-sequence {
          frame #0 {
            n257 = property on="Pane" class="Pane"("Origin"=T8 {"Horizontal"=0, "Vertical"=0}) -> ()  [unwired: 2 in, 2 out]
            n258 = shared-variable-read(refnum<k21> "ni.var.psp://z004551/CDL0100 ReadWriteTags/HMI_BAS_Proc1_AddDIVolume" ("shared variable refnum in"), FALSE) -> (w432:bool)  [unwired: 1 in, 3 out]
            n259 = shared-variable-read(refnum<k21> "ni.var.psp://z004551/CDL0100 ReadWriteTags/HMI_Enable_BTnk1_Pump" ("shared variable refnum in"), FALSE) -> (w429:bool)  [unwired: 1 in, 3 out]
            n260 = shared-variable-read(refnum<k21> "ni.var.psp://z004551/CDL0100 ReadWriteTags/HMI_BAS_Proc1_DI_Setpnt" ("shared variable refnum in"), 0.0) -> (w428:dbl)  [unwired: 1 in, 3 out]
            n261 = shared-variable-read(refnum<k21> "ni.var.psp://z004551/CDL0100 ReadWriteTags/HMI_BAS_TNK1_P_Setpoint" ("shared variable refnum in"), 0.0) -> (w425:dbl)  [unwired: 1 in, 3 out]
            n262 = local write "Add DI Water"(w432) -> ()
            n263 = local write "Enable Main Pump"(w429) -> ()
            n264 = local write "Liters DI to Add"(w428) -> ()
            n265 = local write "Supply Pressure (kPa)"(w425) -> ()
          }
          frame #1 {
            n266 = shared-variable-read(refnum<k21> "ni.var.psp://z004551/CDL0100 ReadWriteTags/HMI_BAS_Tank1_TControl_Enable" ("shared variable refnum in"), FALSE) -> (w449:bool)  [unwired: 1 in, 3 out]
            n267 = shared-variable-read(refnum<k21> "ni.var.psp://z004551/CDL0100 ReadWriteTags/HMI_Proc1_OxFlow_SetPnt" ("shared variable refnum in"), 0.0) -> (w440:dbl)  [unwired: 1 in, 3 out]
            n268 = shared-variable-read(refnum<k21> "ni.var.psp://z004551/CDL0100 ReadWriteTags/HMI_Proc1_Run_OxideSys" ("shared variable refnum in"), FALSE) -> (w443:bool)  [unwired: 1 in, 3 out]
            n269 = shared-variable-read(refnum<k21> "ni.var.psp://z004551/CDL0100 ReadWriteTags/HMI_Proc1_CuOxideAddAmnt" ("shared variable refnum in"), 0.0) -> (w437:dbl)  [unwired: 1 in, 3 out]
            n270 = shared-variable-read(refnum<k21> "ni.var.psp://z004551/CDL0100 ReadWriteTags/HMI_BAS_TNK1_T_Setpoint" ("shared variable refnum in"), 0.0) -> (w446:dbl)  [unwired: 1 in, 3 out]
            n271 = local write "Enable T-Control"(w449) -> ()
            n272 = local write "Flow to Reactor (L/min)"(w440) -> ()
            n273 = local write "Enable Oxide Reactor"(w443) -> ()
            n274 = local write "Temperature Setpoint"(w446) -> ()
            n275 = local write "CuOAddAmount"(w437) -> ()
          }
          frame #2 {
            n276 = shared-variable-read(refnum<k21> "ni.var.psp://z004551/CDL0100 ReadWriteTags/HMI_Dose_SPS_Proc1" ("shared variable refnum in"), FALSE) -> (w459:bool)  [unwired: 1 in, 3 out]
            n277 = shared-variable-read(refnum<k21> "ni.var.psp://z004551/CDL0100 ReadWriteTags/HMI_UCON_Amount_Proc1" ("shared variable refnum in"), 0.0) -> (w452:dbl)  [unwired: 1 in, 3 out]
            n278 = shared-variable-read(refnum<k21> "ni.var.psp://z004551/CDL0100 ReadWriteTags/HMI_Dose_UCON_Proc1" ("shared variable refnum in"), FALSE) -> (w453:bool)  [unwired: 1 in, 3 out]
            n279 = shared-variable-read(refnum<k21> "ni.var.psp://z004551/CDL0100 ReadWriteTags/HMI_BAS_Proc1_Tank_SG" ("shared variable refnum in"), 1.0) -> (w464:dbl)  [unwired: 1 in, 3 out]
            n280 = shared-variable-read(refnum<k21> "ni.var.psp://z004551/CDL0100 ReadWriteTags/HMI_SPS_Amount_Proc1" ("shared variable refnum in"), 0.0) -> (w458:dbl)  [unwired: 1 in, 3 out]
            n281 = local write "Trig SPS Proc 1"(w459) -> ()
            n282 = local write "UCON Proc 1"(w452) -> ()
            n283 = local write "Trig UCON Proc 1"(w453) -> ()
            n284 = local write "Specific Gravity"(w464) -> ()
            n285 = local write "SPS Proc 1"(w458) -> ()
          }
          frame #3 {
            n286 = shared-variable-read(refnum<k21> "ni.var.psp://z004551/CDL0100 ReadWriteTags/HMI_BAS_Proc1_Level_Setpnt" ("shared variable refnum in"), 0.0) -> (w467:dbl)  [unwired: 1 in, 3 out]
            n287 = shared-variable-read(refnum<k21> "ni.var.psp://z004551/CDL0100 ReadWriteTags/HMI_BAS_Proc1_Level_Auto" ("shared variable refnum in"), FALSE) -> (w470:bool)  [unwired: 1 in, 3 out]
            n288 = shared-variable-read(refnum<k21> "ni.var.psp://z004551/CDL0100 ReadWriteTags/HMI_Acid_Amount_Proc1" ("shared variable refnum in"), 0.0) -> (w473:dbl)  [unwired: 1 in, 3 out]
            n289 = shared-variable-read(refnum<k21> "ni.var.psp://z004551/CDL0100 ReadWriteTags/HMI_Leveler_Amount_Proc1" ("shared variable refnum in"), 0.0) -> (w479:dbl)  [unwired: 1 in, 3 out]
            n290 = shared-variable-read(refnum<k21> "ni.var.psp://z004551/CDL0100 ReadWriteTags/HMI_Dose_Acid_Proc1" ("shared variable refnum in"), FALSE) -> (w474:bool)  [unwired: 1 in, 3 out]
            n291 = shared-variable-read(refnum<k21> "ni.var.psp://z004551/CDL0100 ReadWriteTags/HMI_Dose_Leveler_Proc1" ("shared variable refnum in"), FALSE) -> (w480:bool)  [unwired: 1 in, 3 out]
            n292 = local write "Auto Level Main Tank"(w467) -> ()
            n293 = local write "LEV Proc 1"(w479) -> ()
            n294 = local write "Trig Level Proc1"(w480) -> ()
            n295 = local write "Sulfuric Proc 1"(w473) -> ()
            n296 = local write "Trig Sulfuric Proc1"(w474) -> ()
            n297 = local write "Enable DI Auto Top-up"(w470) -> ()
          }
        }
      }
      frame "Exit" {
        # "Destroy message queue >> this will halt the UI event handler loop"
        # "Stop the VI\n>> Perform any cleanup tasks in this message case.\n>> Clear display before closing."
        n298 = call <vilib>:"Destroy Message Queue.vi"("message queue in"=w486, "error in"=w487) -> ("error out"=w485:errorcluster)  [unwired: 11 in, 2 out]
        n299 = local write "status"("" ("Status")) -> ()
      }
      frame "---------- Application Operations ----------" {
        # "Dummy case to add a seperator in the Case Structure menu"
      }
      frame "Write_Tag" {
        n300 = call-poly <vilib>:"Write Message.vi"("error in"=w493, "data"=w491, "name"="WriteTag", "connection info in"=w490) -> ("error out"=w492:errorcluster)  [unwired: 6 in, 1 out]
      }
      frame "DisplayLastHr" {
        n301 = call "Trace Variable 1 hour Popup.vi"("Tag"=w496) -> ()  [unwired: 11 in]
      }
    }
  }
  n302 = call-poly <vilib>:"Get Connection Reference.vi"("error in"=w4, "connection info in"=w5) -> ("error out"=w8:errorcluster, "connection ID out"=w7:refnum<k5>)  [unwired: 8 out]
  n303 = TCP Close Connection(connection ID=w7, error in (no error)=w8) -> (error out=w10:errorcluster)  [unwired: 2 out]
  n304 = call <vilib>:"Error to Warning.vi"("1st Error to Convert"=w9, "error in"=w10) -> ("warning out"=w6:errorcluster)  [unwired: 3 in, 10 out]
  n305 = call <vilib>:"Simple Error Handler.vi"("error in (no error)"=w6) -> ()  [unwired: 4 in, 5 out]
